vi "Create DIT from Hash value & PK.vi"(7 "Public Key (Hex)":string, 8 "error in (no error)":errorcluster, 9 "n (Hex)":string="ÿÿÿÿ", 10 "Private Key (Hex)":string, 11 "Hash value":string="ÿÿÿÿ") -> (0 "error out":errorcluster, 2 "DIT":string="ÿÿÿÿ")   [LabVIEW 2012]
doc: "Creates a data integrity tag (DIT) from a hash value, privite key (PvK), public key (PbK) and n. Uses RSA algorithm, where coded hash string C = B^e mod(n), where\nB = hash value\ne = PK.\n\nFormat of tag\n<DIT><Coded Hash=xxxxx><Public=xxxxx><n=xxxxx></DIT>\n\nNote - the xxxx values are not byte string arrays but the ACSII equivalent (two characters used for each byte)."
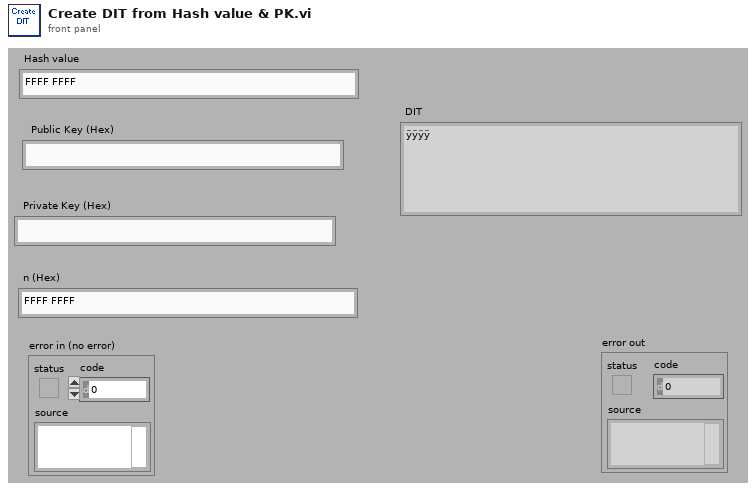
[diagram p1: front panel]
types:
  T1 = typedef "Large number - U8 array.ctl" = u8[]
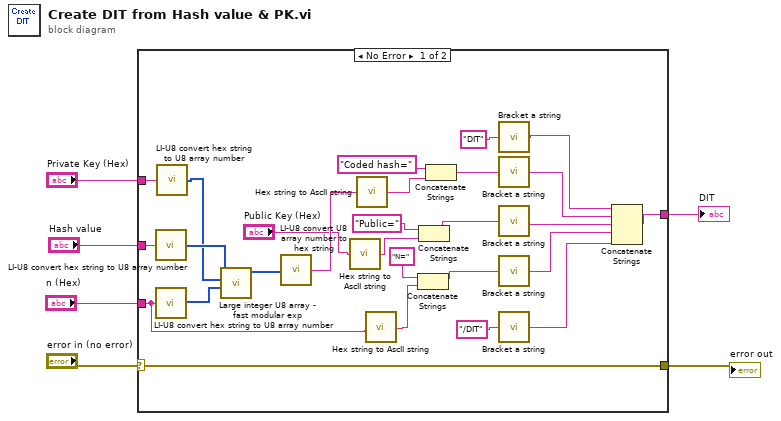
[diagram p0: block diagram]
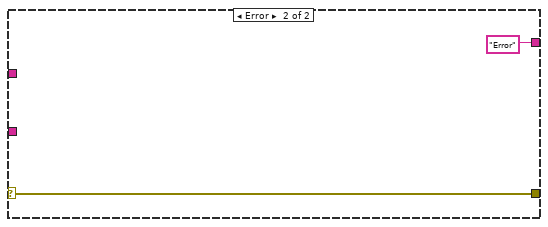
[diagram p2: hidden frame]
diagram:
  n1 = case shown="No Error" "error in (no error)" {
    selector: "error in (no error)" -> [w27 w35]
    tunnel: "n (Hex)" -> [w12 _]
    tunnel: [w27 w35] -> w4
    tunnel: "Private Key (Hex)" -> [w33 _]
    tunnel: "Hash value" -> [w32 _]
    tunnel: [w13 "Error"] -> w1
    frame No Error {
      n2 = call "LI-U8 convert hex string to U8 array number .vi"("hex string (MSD 1st)"=w32) -> ("Large number -U8"=w31:T1)  [unwired: 4 out]
      n3 = call "LI-U8 convert hex string to U8 array number .vi"("hex string (MSD 1st)"=w12) -> ("Large number -U8"=w29:T1)  [unwired: 4 out]
      n4 = call "LI-U8 convert hex string to U8 array number .vi"("hex string (MSD 1st)"=w33) -> ("Large number -U8"=w30:T1)  [unwired: 4 out]
      n5 = call "Large integer U8 array - fast modular exp.vi"("n (LI_U8)"=w29, "Exponent e (LI-U8)"=w30, "B (LI-U8)"=w31) -> ("B^e mod n"=w28:T1)  [unwired: 8 out]
      n6 = call "LI-U8 convert U8 array number to hex string.vi"("Large number -U8"=w28) -> ("hex string (MSD 1st)"=w10:string)  [unwired: 4 out]
      n7 = call "Hex string to AscII string.vi"("hex String"="Public Key (Hex)") -> ("ASCII string"=w7:string)  [unwired: 4 out]
      n8 = call "Hex string to AscII string.vi"("hex String"=w10) -> ("ASCII string"=w9:string)  [unwired: 4 out]
      n9 = call "Hex string to AscII string.vi"("hex String"=w12) -> ("ASCII string"=w11:string)  [unwired: 4 out]
      n10 = Concatenate Strings("N=" ("string"), w11) -> (w19:string)
      n11 = Concatenate Strings("Public=" ("string"), w7) -> (w20:string)
      n12 = Concatenate Strings("Coded hash=" ("string"), w9) -> (w23:string)
      n13 = call "Bracket a string.vi"("String"="DIT") -> ("<string>"=w18:string)  [unwired: 4 out]
      n14 = call "Bracket a string.vi"("String"=w23) -> ("<string>"=w17:string)  [unwired: 4 out]
      n15 = call "Bracket a string.vi"("String"=w20) -> ("<string>"=w16:string)  [unwired: 4 out]
      n16 = call "Bracket a string.vi"("String"=w19) -> ("<string>"=w15:string)  [unwired: 4 out]
      n17 = call "Bracket a string.vi"("String"="/DIT") -> ("<string>"=w14:string)  [unwired: 4 out]
      n18 = Concatenate Strings(w18, w17, w16, w15, w14) -> (w13:string)
    }
    frame Error {
    }
  }
  "error out" <- w4
  "DIT" <- w1
